vi "Fluke 2625A buffer Read.vi"(8 "error out":errorcluster, 11 "VISA resource name out":refnum<visa-resource-name>) -> (0 "error out 2":errorcluster, 2 "read buffer":string, 3 "VISA resource name out 2":refnum<visa-resource-name>)   [LabVIEW 2013, in "Fluke 2625A.lvlib"]
uses:
  <instrlib>/Fluke 2625A/Fluke 2625A.lvlib
panel:
  out "String Contains?":bool
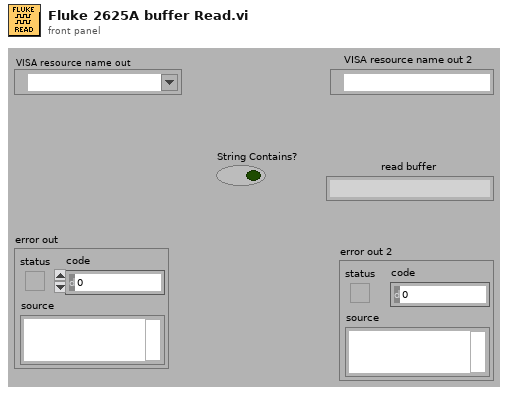
[diagram p1: front panel]
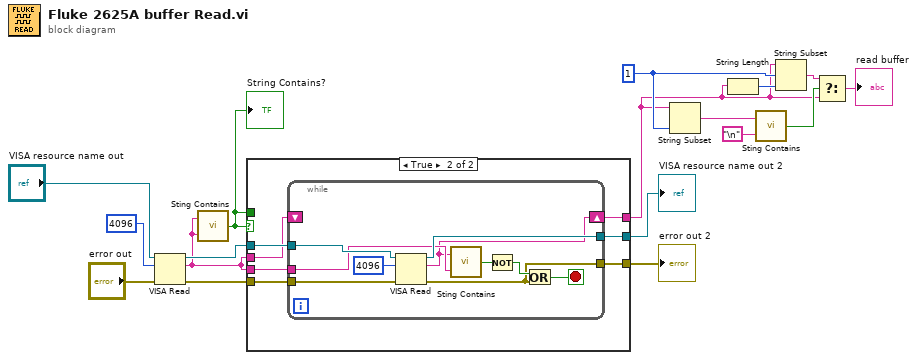
[diagram p0: block diagram]
diagram:
  w10 = 1 ("length (rest)")
  n1 = VISA Read(VISA resource name="VISA resource name out", byte count=u32 4096, error in (no error)="error out") -> (VISA resource name out=w6:refnum<visa-resource-name>, read buffer=w4:string, error out=w5:errorcluster)  [unwired: 1 out]
  n2 = call "Sting Contains.vi"("Expression to evaluate"=w4, "Input String"=w4) -> ("Boolean"=w14:bool)
  "String Contains?" <- w14
  n3 = case shown="True" w14 {
    tunnel: w14 -> [_ _]
    tunnel: w6 -> [w20 w27]
    tunnel: [w20 w26] -> w2
    tunnel: w5 -> [w19 w25]
    tunnel: [w19 w24] -> w1
    tunnel: w4 -> [w18 w23]
    tunnel: [w18 w22] -> w7
    tunnel: w4 -> [_ w21]
    frame False {
    }
    frame True {
      n4 = while {
        tunnel: w27 -> [w37]
        tunnel: [w36] -> w26
        tunnel: w25 -> [w35]
        tunnel: [w33] -> w24
        shift-right: [w28] -> w22
        shift-left: w23 -> [_]
        tunnel: w21 -> [w30]
        stop <- w32 stop-if-true
        n5 = VISA Read(VISA resource name=w37, byte count=u32 4096, error in (no error)=w35) -> (VISA resource name out=w36:refnum<visa-resource-name>, read buffer=w28:string, error out=w33:errorcluster)  [unwired: 1 out]
        n6 = call "Sting Contains.vi"("Expression to evaluate"=w30, "Input String"=w28) -> ("Boolean"=w29:bool)
        n7 = Not(x=w29) -> (.not. x?=w34:bool)
        n8 = Or(x=w34, y=w33) -> (x .or. y?=w32:bool)
      }
    }
  }
  "error out 2" <- w1
  "VISA resource name out 2" <- w2
  n9 = String Subset(string=w7, length (rest)=w10) -> (substring=w9:string)  [unwired: 1 in]
  n10 = String Length(string=w7) -> (length=w8:i32)
  n11 = call "Sting Contains.vi"("Expression to evaluate"="\n", "Input String"=w9) -> ("Boolean"=w12:bool)
  n12 = String Subset(string=w7, offset (0)=w10, length (rest)=w8) -> (substring=w11:string)
  n13 = Select(t=w11, s=w12, f=w7) -> (s? t:f=→"read buffer":string)
